vi "get Clock State.vi"(11 "Clock Generator in":refnum<class "IO.lvclass">) -> (3 "Current State":bool)   [LabVIEW 2021, in "IO.lvclass"]
uses:
  IO.lvclass
  IO.lvclass/IO.ctl
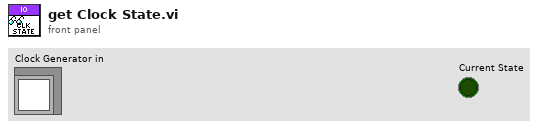
[diagram p1: front panel]
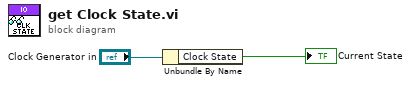
[diagram p0: block diagram]
diagram:
  n1 = Unbundle By Name("Clock Generator in") -> ("Clock State"=→"Current State":bool)
